vi "Get Plot to Fit.vi"(0 "XYGraph in":T3, 9 "Plot Index":i32, 11 "error in (no error)":errorcluster, 12 "Clip Plot? (True)":bool=TRUE) -> (1 "Plot clipped?":bool, 3 "(Clipped) Plot Range":T2, 4 "Full Plot":T1, 6 "Clipped Plot":T1, 10 "Plot Name":string, 13 "Plot Interpolation":u8, 14 "Plot Color":u32, 15 "error out":errorcluster)   [LabVIEW 2021, in "Fits.lvlib"]
uses:
  Fits.lvlib
  Graphs/XY Graph/XY Graph Refnum.ctl
  Graphs/Plot Range.ctl
  Graphs/XY Graph/XY Graph Plot Data.ctl
  Graphs/XY Graph/XY Graph Add-Ons.lvlib
  Graphs/Graphs.lvlib
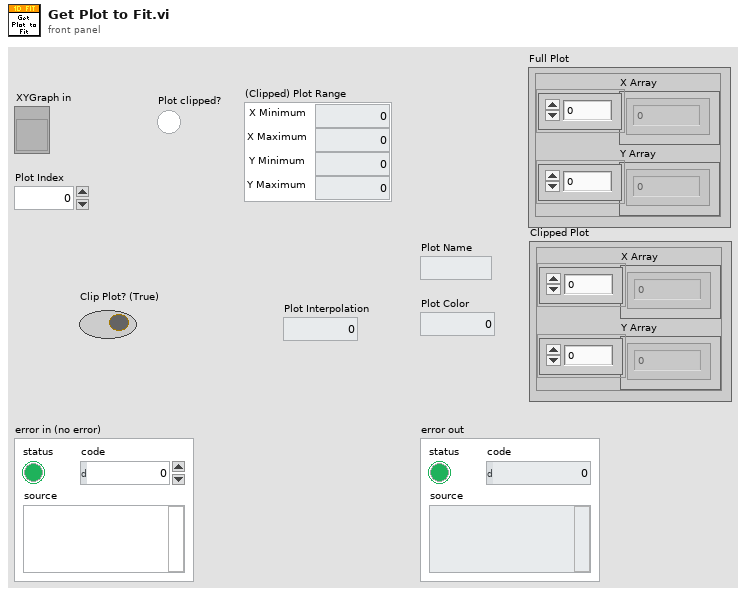
[diagram p1: front panel]
types:
  T1 = typedef "XY Graph Add-Ons.lvlib/XY Graph Plot Data.ctl" = cluster{"X Array":dbl[], "Y Array":dbl[]}
  T2 = typedef "Graphs.lvlib/Plot Range.ctl" = cluster{"X Minimum":dbl, "X Maximum":dbl, "Y Minimum":dbl, "Y Maximum":dbl}
  T3 = typedef "XY Graph Add-Ons.lvlib/XY Graph Refnum.ctl" = refnum<vi>
  T4 = typedef "Histogram Window.lvlib/Histogram Bin Position.ctl" = enum16{"Left", "Center", "Right"}
  T5 = cluster{"X Array out":dbl[], "Y Array out":dbl[]}
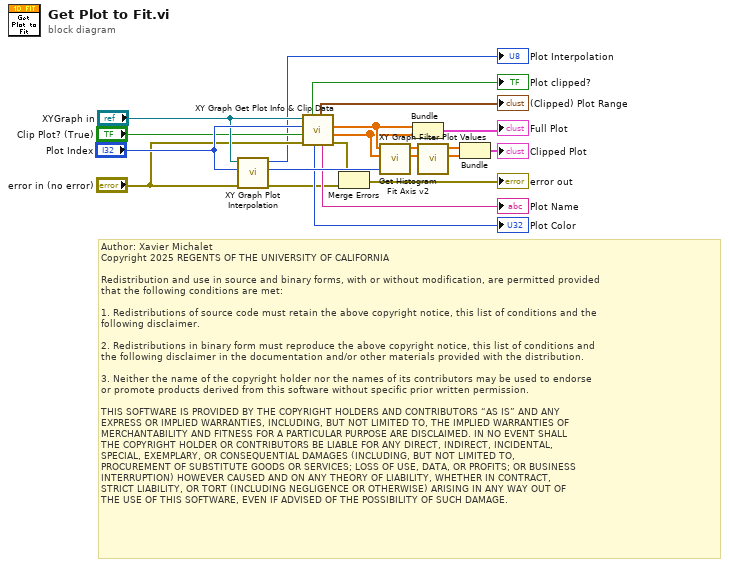
[diagram p0: block diagram]
diagram:
  # "Author: Xavier Michalet\nCopyright 2025 REGENTS OF THE UNIVERSITY OF CALIFORNIA\n\nRedistribution and use in source and binary forms, with or without modification, are permitted provided\nthat the following conditions are met:\n\n1. Redistributions of source code must retain the above copyright notice, this list of conditions and the\nfollowing disclaimer.\n\n2. Redistributions in binary form must reproduce the above copyright notice, this list of conditions and\nthe following disclaimer in the documentation and/or other materials provided with the distribution.\n\n3. Neither the name of the copyright holder nor the names of its contributors may be used to endorse \nor promote products derived from this software without specific prior written permission.\n\nTHIS SOFTWARE IS PROVIDED BY THE COPYRIGHT HOLDERS AND CONTRIBUTORS “AS IS” AND ANY \nEXPRESS OR IMPLIED WARRANTIES, INCLUDING, BUT NOT LIMITED TO, THE IMPLIED WARRANTIES OF\nMERCHANTABILITY AND FITNESS FOR A PARTICULAR PURPOSE ARE DISCLAIMED. IN NO EVENT SHALL\nTHE COPYRIGHT HOLDER OR CONTRIBUTORS BE LIABLE FOR ANY DIRECT, INDIRECT, INCIDENTAL, \nSPECIAL, EXEMPLARY, OR CONSEQUENTIAL DAMAGES (INCLUDING, BUT NOT LIMITED TO, \nPROCUREMENT OF SUBSTITUTE GOODS OR SERVICES; LOSS OF USE, DATA, OR PROFITS; OR BUSINESS\nINTERRUPTION) HOWEVER CAUSED AND ON ANY THEORY OF LIABILITY, WHETHER IN CONTRACT, \nSTRICT LIABILITY, OR TORT (INCLUDING NEGLIGENCE OR OTHERWISE) ARISING IN ANY WAY OUT OF\nTHE USE OF THIS SOFTWARE, EVEN IF ADVISED OF THE POSSIBILITY OF SUCH DAMAGE."
  n1 = call "XY Graph Plot Interpolation.vi"("error in (no error)"="error in (no error)", "Active Plot"="Plot Index", "XYGraph in"="XYGraph in") -> ("error out"=w11:errorcluster, "Bin Location"=w21:T4, "Plot Interpolation"=→"Plot Interpolation":u8)  [unwired: 6 in]
  n2 = call "XY Graph Get Plot Info & Clip Data.vi"("error in (no error)"="error in (no error)", "Clip Plot? (True)"="Clip Plot? (True)", "Plot index"="Plot Index", "XYGraph Ref in"="XYGraph in") -> ("error out"=w15:errorcluster, "Y Array"=w6:dbl[], "X Array"=w7:dbl[], "Plot Name"=→"Plot Name":string, "Plot Range"=→"(Clipped) Plot Range":T2, "Plot Color"=→"Plot Color":u32, "Plot Clipped?"=→"Plot clipped?":bool)  [unwired: 1 out]
  n3 = Merge Errors(w15, w11) -> (→"error out":errorcluster)
  n4 = call "Get Histogram Fit Axis v2.vi"("Bin Location (Left)"=w21, "Plot Values"=w6, "Plot Axis"=w7) -> ("Ordered Axis Plot Values"=w17:dbl[], "Ordered Plot Axis"=w16:dbl[])  [unwired: 3 in, 4 out]
  n5 = Bundle("X Array"=w7, "Y Array"=w6) -> (→"Full Plot":cluster{"X Array":dbl[], "Y Array":dbl[]})  [unwired: 1 in]
  n6 = call "XY Graph Filter Plot Values.vi"("Y Array in"=w17, "X Array in"=w16) -> ("Y Array out"=w3:dbl[], "X Array out"=w4:dbl[])  [unwired: 7 in, 1 out]
  n7 = Bundle("X Array out"=w4, "Y Array out"=w3) -> (→"Clipped Plot":T5)  [unwired: 1 in]
